vi "SerialRW.vi"(5 "Query?":bool, 6 "error in (no error)":errorcluster, 7 "Delay (ms)":u32=300, 8 "Command":string, 9 "VISA handle":refnum<visa-resource-name>) -> (0 "error out":errorcluster, 2 "Response":string, 3 "Dup. VISA handle":refnum<visa-resource-name>, 4 "TimeoutFlag":bool)   [LabVIEW 2019]
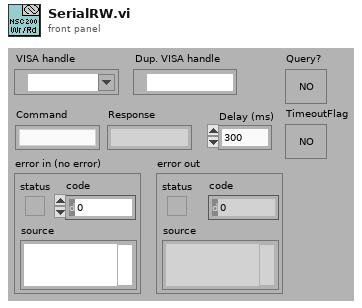
[diagram p1: front panel]
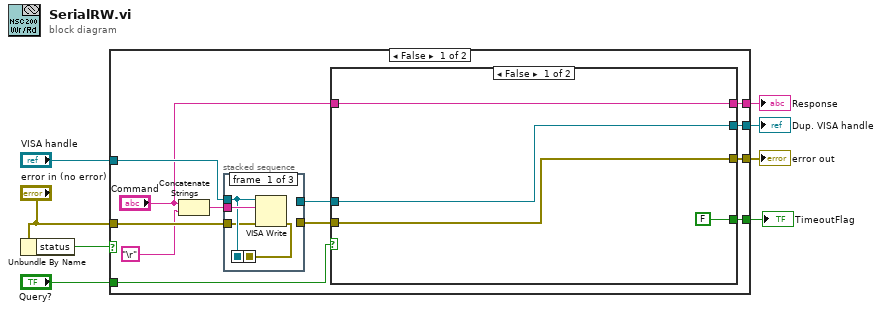
[diagram p0: block diagram]
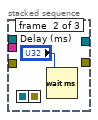
[diagram p2: hidden frame]
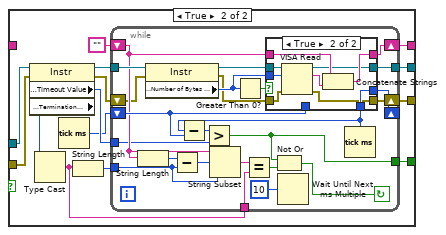
[diagram p4: hidden frame]
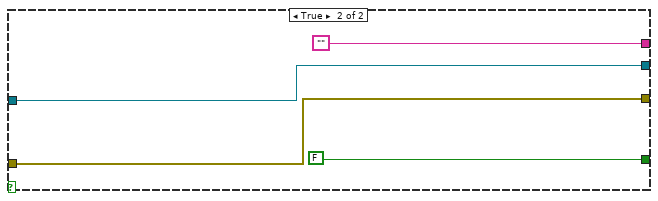
[diagram p6: hidden frame]
diagram:
  n1 = Unbundle By Name("error in (no error)") -> ("status"=w5:bool)
  n2 = case shown="False" w5 {
    tunnel: "VISA handle" -> [w20 w86]
    tunnel: [w16 w86] -> w7
    tunnel: [w15 w85] -> w6
    tunnel: "error in (no error)" -> [w19 w85]
    tunnel: [w14 ""] -> w3
    tunnel: [w13 FALSE] -> w2
    tunnel: "Query?" -> [w11 _]
    frame False {
      n3 = Concatenate Strings("Command", "\r") -> (w12:string)
      n4 = stacked-sequence {
        seq-local: [w23 _ _] -> [_ _ w27]
        seq-local: [w21 _ _] -> [_ _ w26]
        tunnel: w20 -> [w23 _ _]
        tunnel: w12 -> [w24 _ _]
        tunnel: w19 -> [w22 _ _]
        tunnel: [_ _ w27] -> w18
        tunnel: [_ _ w26] -> w17
        frame #0 {
          n5 = VISA Write(VISA resource name=w23, write buffer=w24, error in (no error)=w22) -> (error out=w21:errorcluster)  [unwired: 2 out]
        }
        frame #1 {
          n6 = Wait (ms)(milliseconds to wait="Delay (ms)") -> ()  [unwired: 1 out]
        }
        frame #2 {
        }
      }
      n7 = case shown="False" w11 {
        tunnel: [w30 w35] -> w15
        tunnel: [w31 w36] -> w16
        tunnel: w18 -> [w31 w45]
        tunnel: w17 -> [w30 w44]
        tunnel: [w28 w34] -> w14
        tunnel: [FALSE w32] -> w13
        tunnel: "Command" -> [w28 _]
        frame False {
        }
        frame True {
          n8 = property class="Instr"(reference=w45, error in=w44) -> (reference out=w43:refnum<visa-resource-name>, error out=w42:errorcluster, "General Settings:Timeout Value"=w41:u32, "Message Based Settings:Termination Character"=w39:u8)
          n9 = Type Cast(x=w39) -> (*(type *) &x=w37:string)  [unwired: 1 out]
          n10 = Tick Count (ms)() -> (millisecond timer value=w38:u32)
          n11 = String Length(string=w37) -> (length=w40:i32)
          n12 = while {
            tunnel: w40 -> [w55]
            tunnel: w41 -> [w54]
            tunnel: w43 -> [w69]
            shift-right: [w65] -> w34
            shift-left: "" -> [w56]
            shift-right: [w63] -> _
            shift-left: w38 -> [w62]
            tunnel: w37 -> [w57]
            tunnel: [w51] -> w32
            tunnel: [w50] -> w36
            shift-right: [w49] -> w35
            shift-left: w42 -> [w48]
            stop <- w52 continue-if-true
            n13 = String Length(string=w56) -> (length=w60:i32)
            n14 = property class="Instr"(reference=w69, error in=w48) -> (reference out=w67:refnum<visa-resource-name>, error out=w47:errorcluster, "Serial Settings:Number of Bytes at Serial Port"=w66:u32)
            n15 = Subtract(x=w60, y=w55) -> (x-y=w59:i32)
            n16 = String Subset(string=w56, offset (0)=w59, length (rest)=w55) -> (substring=w58:string)
            n17 = Greater Than 0?(x=w66) -> (x > 0?=w68:bool)
            n18 = Equal?(x=w58, y=w57) -> (x = y?=w53:bool)
            n19 = Wait Until Next ms Multiple(millisecond multiple=u32 10) -> ()  [unwired: 1 out]
            n20 = Tick Count (ms)() -> (millisecond timer value=w64:u32)
            n21 = Subtract(x=w64, y=w62) -> (x-y=w61:u32)
            n22 = Greater?(x=w61, y=w54) -> (0:w51:bool)
            n23 = case shown="True" w68 {
              tunnel: w67 -> [w71 w82]
              tunnel: w66 -> [_ w81]
              tunnel: w56 -> [w73 w79]
              tunnel: [w73 w78] -> w65
              tunnel: w64 -> [_ w77]
              tunnel: [w72 w77] -> w63
              tunnel: w62 -> [w72 _]
              tunnel: [w71 w76] -> w50
              tunnel: w47 -> [w70 w75]
              tunnel: [w70 w74] -> w49
              frame False {
              }
              frame True {
                n24 = VISA Read(VISA resource name=w82, byte count=w81, error in (no error)=w75) -> (VISA resource name out=w76:refnum<visa-resource-name>, read buffer=w80:string, error out=w74:errorcluster)  [unwired: 1 out]
                n25 = Concatenate Strings(w79, w80) -> (w78:string)
              }
            }
            n26 = Not Or(1:w53, 2:w51) -> (0:w52:bool)
          }
        }
      }
    }
    frame True {
    }
  }
  "Dup. VISA handle" <- w7
  "error out" <- w6
  "Response" <- w3
  "TimeoutFlag" <- w2
